vi "读取质控数据.vi"(7 "结束索引记录":timestamp, 8 "错误输入（无错误）":errorcluster, 9 "模式":enum16{"零点核查", "跨度核查"}(ring), 10 "table":string, 11 "起始索引记录":timestamp) -> (0 "错误输出":errorcluster, 3 "data":T1(array[cluster]))   [LabVIEW 2016, in "数据查询.lvlib"]
uses:
  <vilib>/addons/database/Connection.llb/DB Tools Open Connec (String).vi
  <vilib>/addons/database/_DB Variant To Data/Database Variant To Data.xnode
  <vilib>/addons/database/NI_Database_API.lvlib
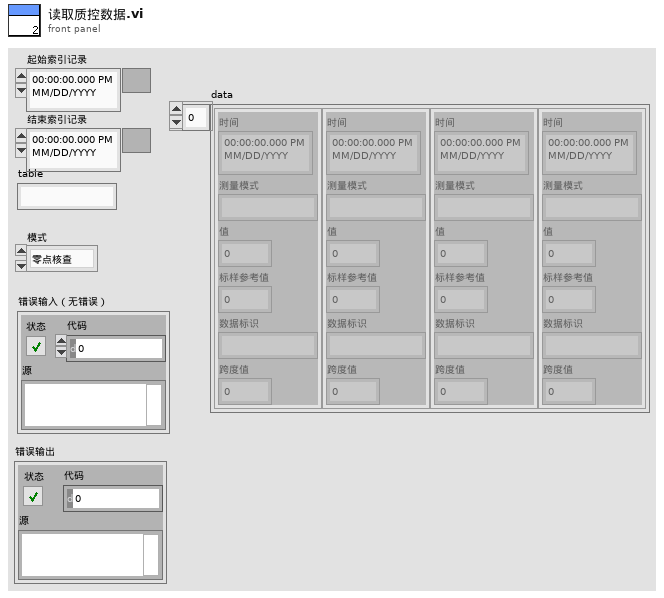
[diagram p1: front panel]
types:
  T1 = cluster{"时间":timestamp, "测量模式":string, "值":sgl, "标样参考值":sgl, "数据标识":string, "跨度值":sgl}[]
  T2 = cluster{"时间":timestamp, "测量模式":string, "值":sgl, "值 2":sgl, "数据标识":string, "值 3":sgl}[]
  T3 = typedef "NI_Database_API.lvlib/Conn ObjectReference.ctl" = refnum<k1>
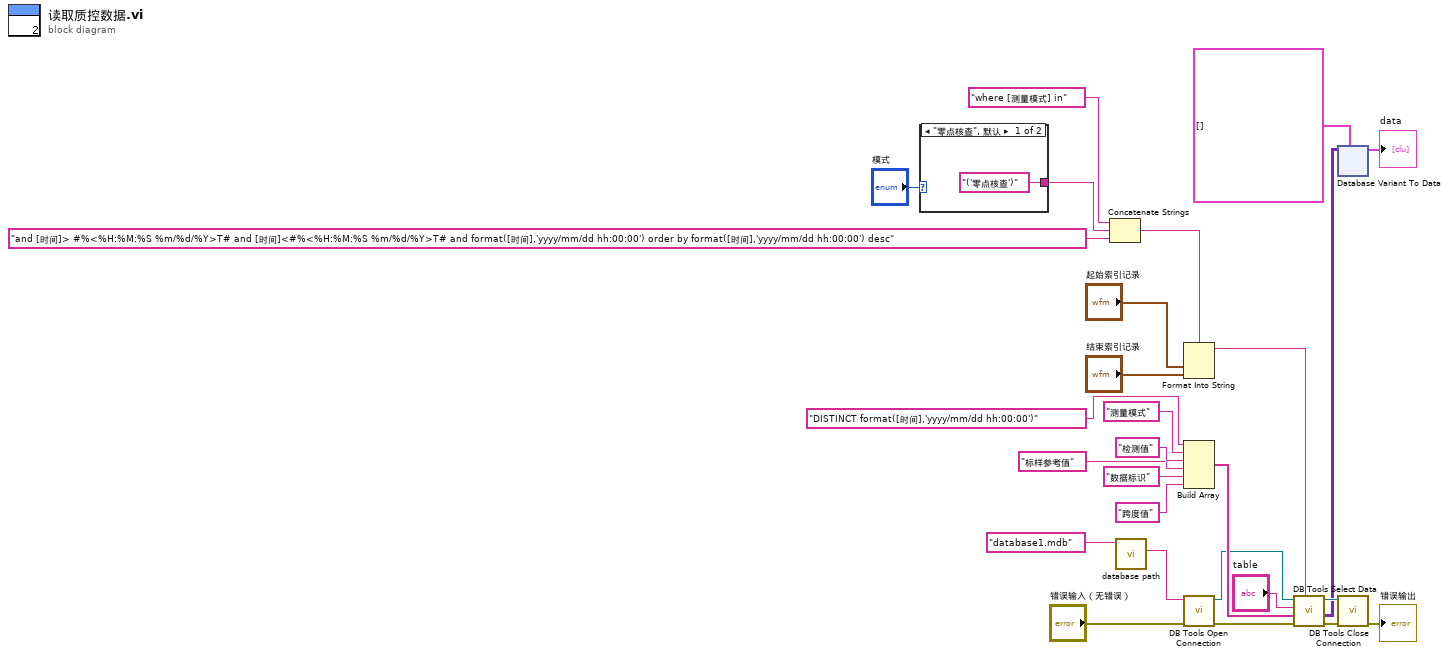
[diagram p0: block diagram]
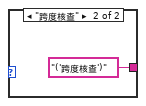
[diagram p2: hidden frame]
diagram:
  n1 = case shown="\"零点核查\", 默认" "模式" {
    tunnel: ["('零点核查')" "('跨度核查')"] -> w6
    frame "零点核查", Default {
    }
    frame "跨度核查" {
    }
  }
  n2 = Concatenate Strings("where [测量模式] in" ("condition"), w6, "and [时间]> #%<%H:%M:%S %m/%d/%Y>T# and [时间]<#%<%H:%M:%S %m/%d/%Y>T# and format([时间],'yyyy/mm/dd hh:00:00') order by format([时间],'yyyy/mm/dd hh:00:00') desc" ("condition")) -> (w5:string)
  n3 = call "database path.vi"("database"="database1.mdb") -> ("Connection information"=w13:string)  [unwired: 9 in, 1 out]
  n4 = Format Into String(format string=w5, "起始索引记录", "结束索引记录") -> (resulting string=w20:string)  [unwired: 2 in, 1 out]
  n5 = Build Array("DISTINCT format([时间],'yyyy/mm/dd hh:00:00')", "测量模式" ("元素"), "检测值" ("元素"), "标样参考值" ("元素"), "数据标识" ("元素"), "跨度值" ("元素")) -> (w16:string[])
  n6 = call-poly <vilib>:"DB Tools Open Connection.vi"("error in (no error)"="错误输入（无错误）", "connection information"=w13) -> ("error out"=w12:errorcluster, "connection reference"=w11:T3)  [unwired: 6 in]
  n7 = call <vilib>:"DB Tools Select Data.vi"("condition"=w20, "error in (no error)"=w12, "columns"=w16, "table"="table", "connection reference"=w11) -> ("error out"=w24:errorcluster, "data"=w22:variant[][], "connection reference out"=w23:T3)  [unwired: 1 in]
  n8 = xnode "Database Variant To Data"("database variant"=w22, "type"=T2 []) -> ("data"=→"data":T2)  [unwired: 1 in, 1 out]
  n9 = call <vilib>:"DB Tools Close Connection.vi"("error in (no error)"=w24, "connection reference"=w23) -> ("error out"=→"错误输出":errorcluster)  [unwired: 5 in]
